vi "Get Library Refnum.vi"(11 "error in (no error)":errorcluster) -> (4 "Library Refnum":refnum<vi>, 6 "Project:Open":refnum<vi>, 15 "error out":errorcluster)   [LabVIEW 2021, in "Migrator.lvlib"]
uses:
  Migrator.lvlib
  Migrator Reusables/Migrator Reusables.lvlib
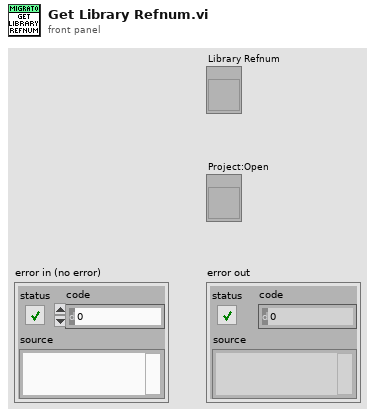
[diagram p1: front panel]
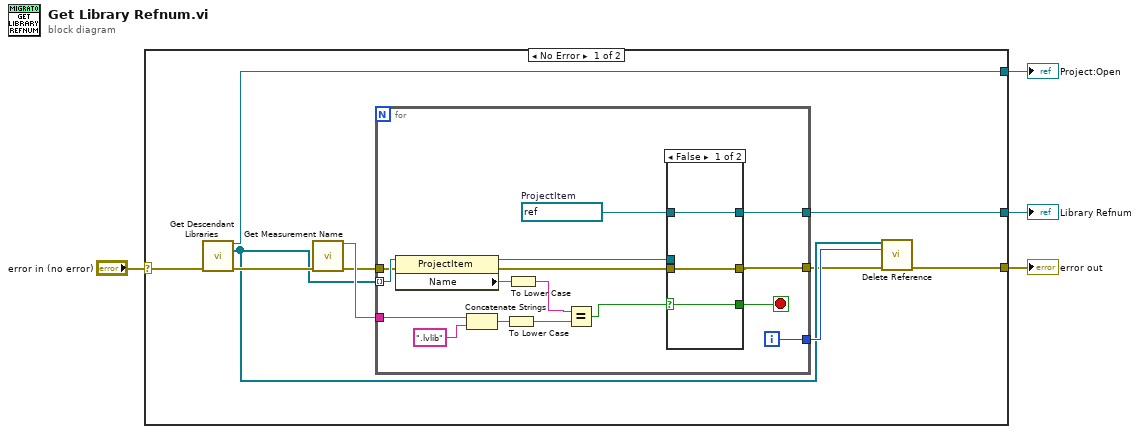
[diagram p0: block diagram]
diagram:
  n1 = case shown="No Error" "error in (no error)" {
    selector: "error in (no error)" -> [w12 w37]
    tunnel: [w14 _] -> w4
    tunnel: [w5 w37] -> w3
    tunnel: [w13 _] -> w2
    frame No Error {
      n2 = call "Get Descendant Libraries.vi"("error in (no error)"=w12) -> ("Project out"=w13:refnum<vi>, "All Descendents"=w7:refnum<vi>[], "error out"=w10:errorcluster)  [unwired: 12 in]
      n3 = call "Get Measurement Name.vi"("error in (no error)"=w10) -> ("Name Out"=w11:string, "error out"=w9:errorcluster)  [unwired: 13 in]
      n4 = for {
        tunnel: w7 -> [w30] mode=indexing
        tunnel: [w23] -> w14
        tunnel: [w22] -> w6
        tunnel: w11 -> [w21]
        tunnel: w9 -> [w20]
        tunnel: [w15] -> w8
        i -> [w15]
        stop <- w24 stop-if-true
        w27 = refnum<vi> refnum  # ProjectItem
        n5 = property class="ProjectItem"(reference=w30, error in=w20) -> (reference out=w26:refnum<vi>, error out=w25:errorcluster, "Name"=w29:string)
        n6 = Concatenate Strings(w21, ".lvlib" ("string")) -> (w19:string)
        n7 = To Lower Case(string=w19) -> (all lower case string=w16:string)
        n8 = To Lower Case(string=w29) -> (all lower case string=w17:string)
        n9 = Equal?(x=w17, y=w16) -> (x = y?=w28:bool)
        n10 = case shown="False" w28 {
          selector: w28 -> [w32 w35]
          tunnel: w26 -> [_ w36]
          tunnel: [w31 w34] -> w22
          tunnel: [w33 w36] -> w23
          tunnel: w27 -> [w33 _]
          tunnel: [w32 w35] -> w24
          tunnel: w25 -> [w31 w34]
          frame False {
          }
          frame True {
          }
        }
      }
      n11 = call "Delete Reference.vi"("All Descendents"=w7, "Numeric"=w8, "error in (no error)"=w6) -> ("error out"=w5:errorcluster)  [unwired: 12 in]
    }
    frame Error {
    }
  }
  "Library Refnum" <- w4
  "error out" <- w3
  "Project:Open" <- w2
